vi "WDAV.vi"(8 "error in (no error)":errorcluster, 9 "local file path":path, 10 "remote path with slash files":string, 11 "target ip":string) -> (0 "error out":errorcluster)   [LabVIEW 2019]
uses:
  <vilib>/WebDAVClient/Simple Put File.vi
  <vilib>/WebDAVClient/NI_WebDAV.lvlib
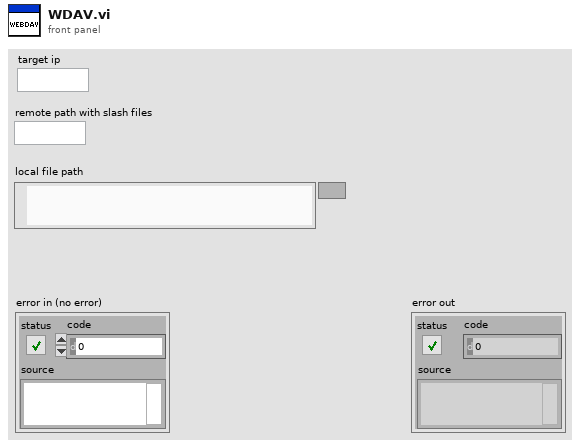
[diagram p1: front panel]
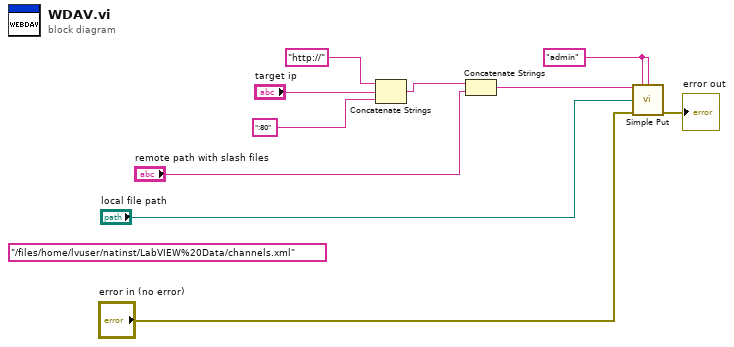
[diagram p0: block diagram]
diagram:
  (unwired) "/files/home/lvuser/natinst/LabVIEW%20Data/channels.xml" ("string")
  w6 = "admin" ("username")
  n1 = Concatenate Strings("http://" ("string"), "target ip", ":80" ("string")) -> (w3:string)
  n2 = Concatenate Strings(w3, "remote path with slash files") -> (w4:string)
  n3 = call-poly <vilib>:"Simple Put.vi"("file uri"=w4, "username"=w6, "password"=w6, "local file path"="local file path", "error in (no error)"="error in (no error)") -> ("error out"=→"error out":errorcluster)  [unwired: 9 in, 1 out]
